vi "VAC_Measure_3.vi"() -> ()   [LabVIEW 2018]
doc: "Read one the value of one analog channel from a LINX device."
uses:
  <vilib>/MakerHub/LINX/Public/Peripherals/Digital/Digital Write N Chans.vi
  <vilib>/MakerHub/LINX/Public/Peripherals/Digital/Digital Write 1 Chan.vi
  <vilib>/MakerHub/LINX/Public/Peripherals/Analog/Analog Read N Chans.vi
  <vilib>/MakerHub/LINX/Private/Local IO/LinxDigitalWrite.vi
  <vilib>/MakerHub/LINX/Public/Utilities/Check Channel.vi
  <vilib>/MakerHub/LINX/Private/Local IO/LinxAnalogRead.vi
  <vilib>/MakerHub/LINX/Public/Utilities/Open Serial.vi
  <vilib>/MakerHub/LINX/Private/Utilties/Generate Error.vi
  <vilib>/MakerHub/LINX/LMH-LINX.lvlib
  LW/LIRA_toolbox.lvlib
panel:
  in  "Каналы разрядки":u8[](array[numeric])
  in  "Каналы зарядки":u8[](array[numeric])
  out "Напряжение":T1(graph)
  out "Ток":T1(graph)
  out "Напряжение":dbl[](array[numeric])
  out "Сила тока":dbl[](array[numeric])
  in  "Каналы чтения напряжения":u8[](array[numeric])
  in  "Каналы чтения тока":u8[](array[numeric])
  in  "Boolean":bool
  in  "Макс напряжение":dbl
  in  "Канал шторки":u8
  in  "Старт программы":bool
  in  "Напряжение":T2={"Измеряемая величина"="U", "единицы измерения"="В", "Ширина строки (в символах)"="16", "Количество знаков после запятой"="2"}
  in  "Сила тока":T2={"Измеряемая величина"="I", "единицы измерения"="A", "Ширина строки (в символах)"="16", "Количество знаков после запятой"="2"}
  in  "Количество стрингов":i32=1
  in  "Название файла":string="1"
  in  "Путь к файлу с указанием на случайный txt файл":path=path "I:/Снятие_ВАХ/log/20250902_16_09_1.txt"
  in  "Старт измерений":bool
  out "array of clusters":cluster{"Voltage":dbl, "Voltage":dbl}[](array[cluster])
  out "ВАХ":cluster{"X":dbl, "Y":dbl}[](graph)
  out "Loop Rate (Hz)":u32
  in  "Stop Button":bool
  in  "Serial Port":refnum<visa-resource-name>="COM6"
  # "Панель управления"
  # "LINX Device Settings"
  # "Панель вывода данных на экран"
  # "Панель вывода данных в файл"
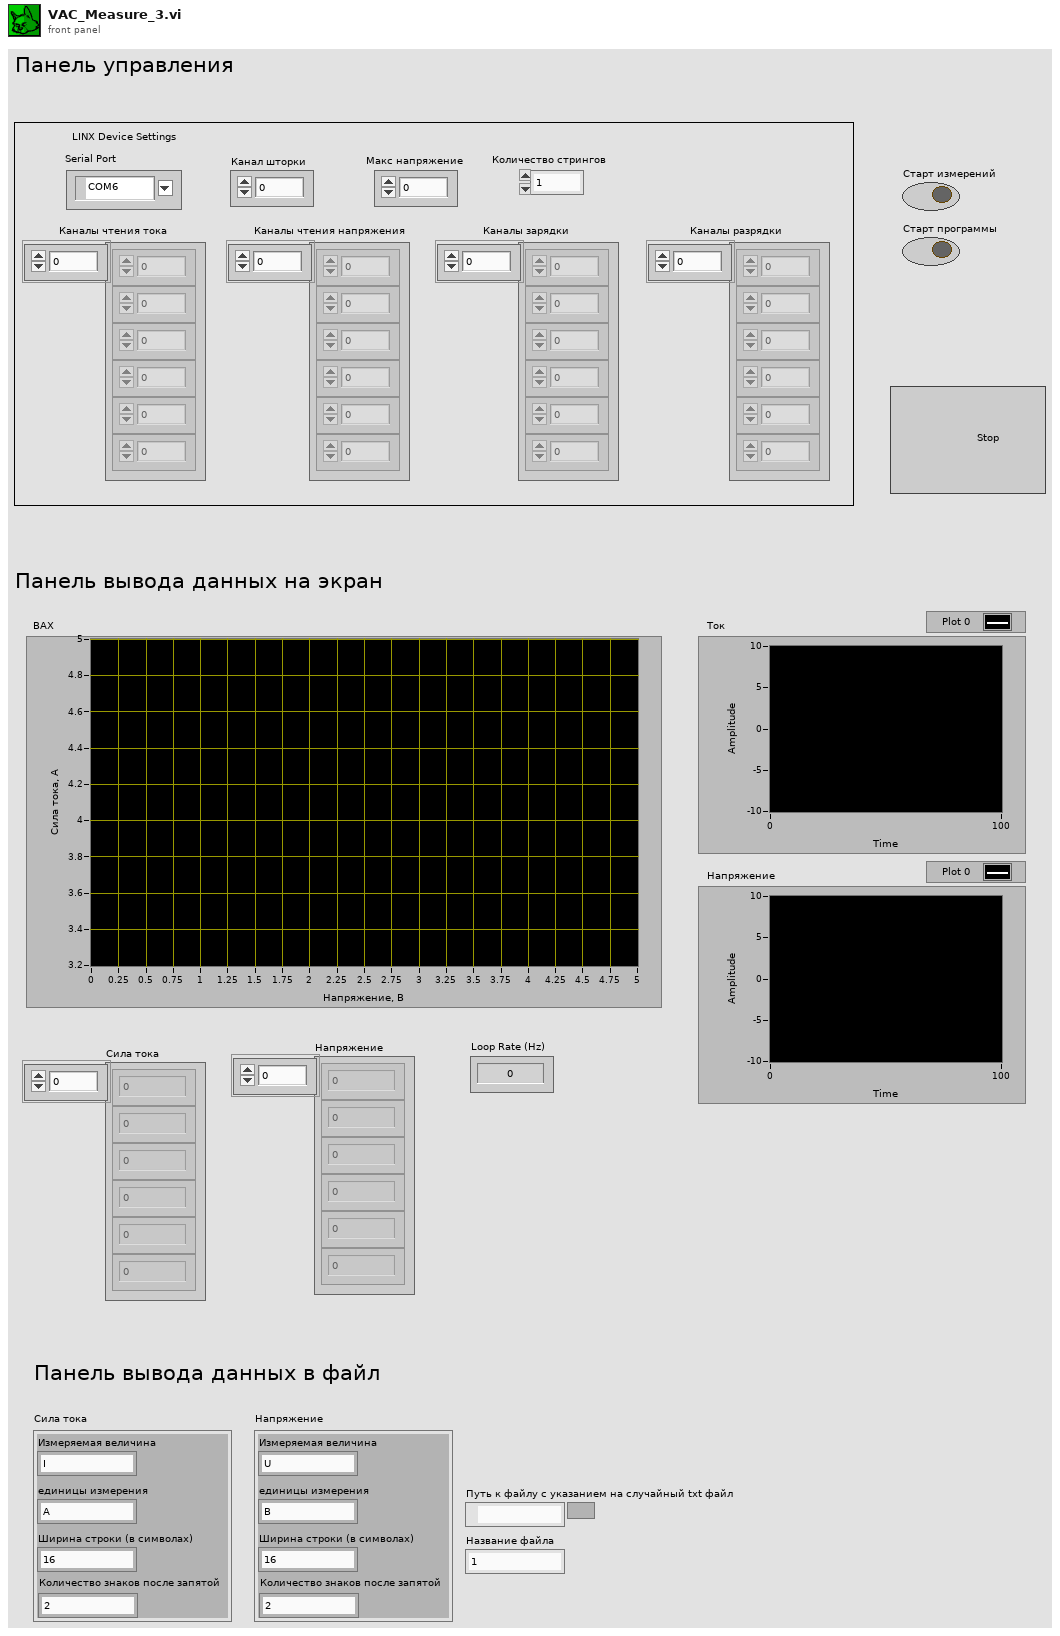
[diagram p1: front panel]
types:
  T1 = cluster{"Voltages[0]":dbl, "Voltages[1]":dbl, "Voltages[2]":dbl, "Voltages[3]":dbl, "Voltages[4]":dbl, "Voltages[5]":dbl, "Voltages[6]":dbl, "Voltages[7]":dbl, "Voltages[8]":dbl}
  T2 = cluster{"Измеряемая величина":string, "единицы измерения":string, "Ширина строки (в символах)":string, "Количество знаков после запятой":string}
  T3 = typedef "LMH-LINX.lvlib/LINX Ref.ctl" = cluster{"IO":T4, "Interface":T5, "LINX Device Config":T6}
  T4 = typedef "LMH-LINX.lvlib/Platform.ctl" = enum16{"Remote", "Local"}
  T5 = typedef "LMH-LINX.lvlib/Interface.ctl" = enum16{"Serial", "TCP"}
  T6 = typedef "LMH-LINX.lvlib/Device.lvlib/LINX Device Config.ctl" = cluster{"Interface":T5, "COM Port":refnum<visa-resource-name>, "TCP Configuration":T7, "Device Family":u8, "Device ID":u8, "Device Name":string, "TCP Ref":refnum<k5>, "Channels":T8}
  T7 = typedef "LMH-LINX.lvlib/Device.lvlib/TCP Config.ctl" = cluster{"IP Address":string, "Port":u16}
  T8 = typedef "LMH-LINX.lvlib/Channels.ctl" = cluster{"DI":u8[], "DO":u8[], "AI":u8[], "AO":u8[], "PWM":u8[], "QE":u8[], "UART":u8[], "I2C 2":u8[], "SPI":u8[], "CAN":u8[], "Servo":u8[], "AI Ref (V)":dbl, "AI Resolution (Bits)":u8, "AO Ref (V)":dbl, "AO Resolution (Bits)":u8}
  T9 = cluster{"Numeric Control":dbl, "Numeric Control":dbl}[]
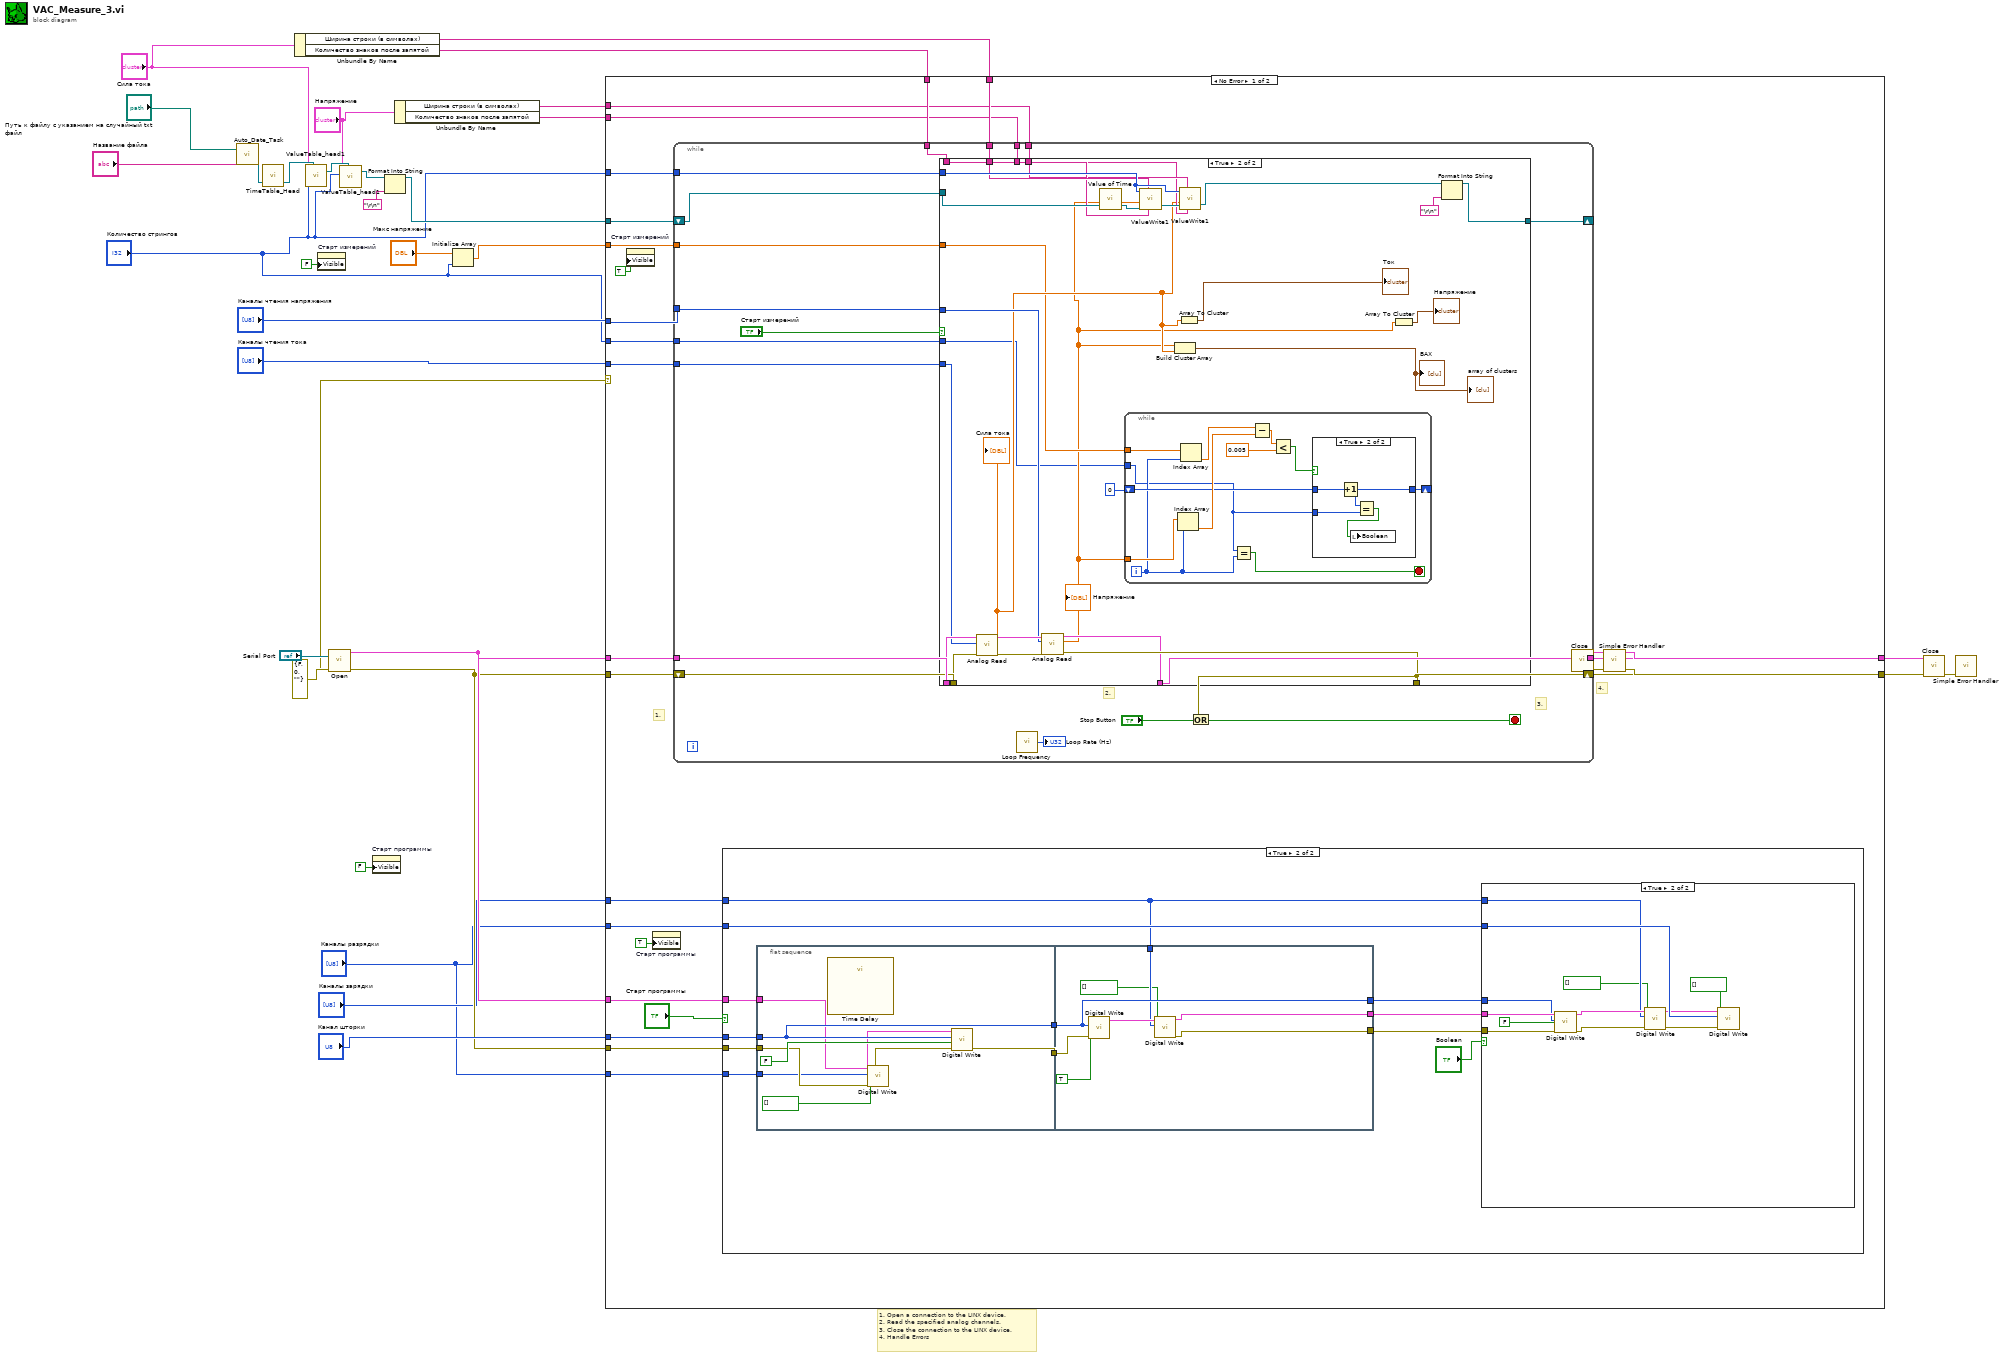
[diagram p0: block diagram]
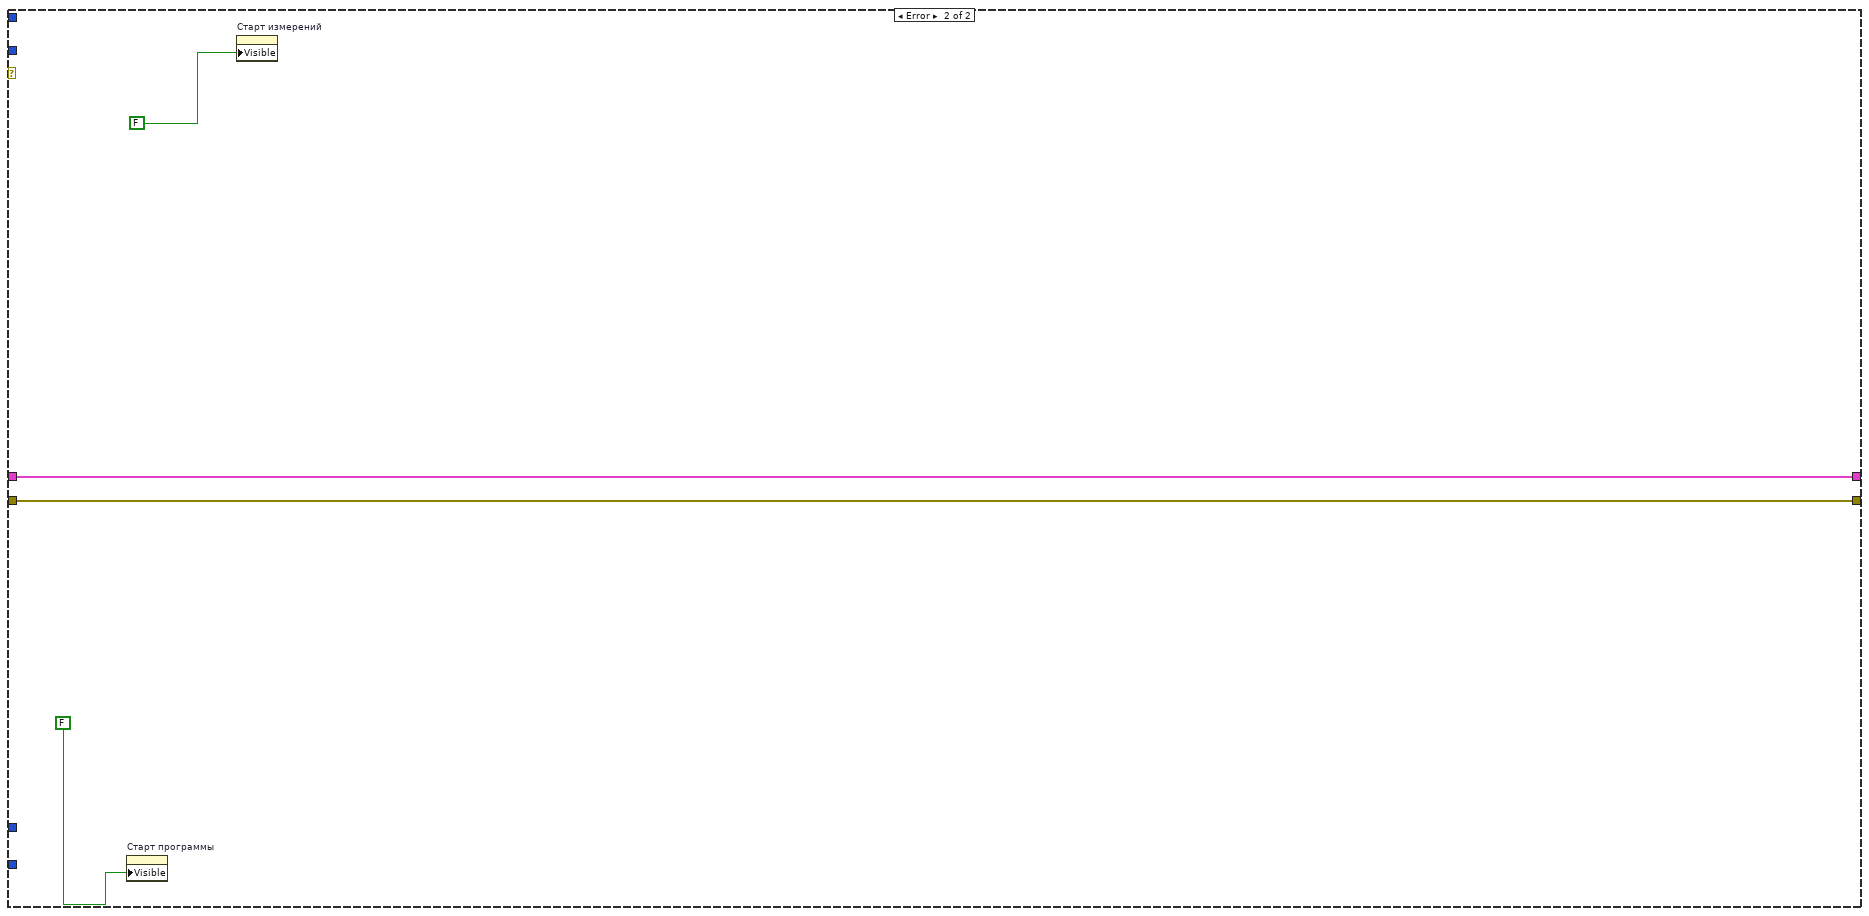
[diagram p6: hidden frame]
diagram:
  # "1. Open a connection to the LINX device.\n2. Read the specified analog channels.\n3. Close the connection to the LINX device.\n4. Handle Errors"
  # "4."
  n1 = call "Auto_Date_Task.vi"("Название файла"="Название файла", "Путь к файлу с указанием на случайный txt файл"="Путь к файлу с указанием на случайный txt файл") -> ("refnum out"=w26:refnum<file>)  [unwired: 1 out]
  n2 = call "TimeTable_Head.vi"("input file"=w26) -> ("output file refnum"=w25:refnum<file>)  [unwired: 1 in, 1 out]
  n3 = Unbundle By Name("Сила тока") -> ("Ширина строки (в символах)"=w22:string, "Количество знаков после запятой"=w21:string)
  n4 = call "ValueTable_head1.vi"("Файл записи"=w25, "Количество датчиков"="Количество стрингов", "Cluster"="Сила тока") -> ("Файл записи 2"=w24:refnum<file>)  [unwired: 3 in, 1 out]
  n5 = property on="Старт измерений" class="Bool (strict)"("Visible"=FALSE) -> ()  [unwired: 2 in, 2 out]
  n6 = call-poly <vilib>:"Open.vi"("Error In"=errorcluster {"status"=FALSE, "code"=0, "source"=""}, "Serial Port"="Serial Port") -> ("Error Out"=w11:errorcluster, "LINX Resource"=w13:T3)  [unwired: 7 in, 1 out]
  n7 = call "ValueTable_head1.vi"("Файл записи"=w24, "Количество датчиков"="Количество стрингов", "Cluster"="Напряжение") -> ("Файл записи 2"=w16:refnum<file>)  [unwired: 3 in, 1 out]
  n8 = property on="Старт программы" class="Bool (strict)"("Visible"=FALSE) -> ()  [unwired: 2 in, 2 out]
  n9 = Format Into String(initial string=w16, "\r\n") -> (resulting string=w15:refnum<file>)  [unwired: 2 in, 1 out]
  n10 = Unbundle By Name("Напряжение") -> ("Ширина строки (в символах)"=w19:string, "Количество знаков после запятой"=w18:string)
  n11 = Initialize Array("Макс напряжение", "Количество стрингов") -> (w7:dbl[])
  n12 = case shown="No Error" w11 {
    tunnel: w13 -> [w55 w165]
    tunnel: w11 -> [w54 w166]
    tunnel: [w53 w165] -> w3
    tunnel: [w52 w166] -> w2
    tunnel: w15 -> [w51 _]
    tunnel: "Количество стрингов" -> [w49 _]
    tunnel: w22 -> [w48 _]
    tunnel: w21 -> [w47 _]
    tunnel: w19 -> [w46 _]
    tunnel: w18 -> [w45 _]
    tunnel: w13 -> [w42 _]
    tunnel: "Канал шторки" -> [w41 _]
    tunnel: w11 -> [w40 _]
    tunnel: "Каналы чтения тока" -> [w39 _]
    tunnel: "Каналы чтения напряжения" -> [w38 _]
    tunnel: w7 -> [w37 _]
    tunnel: "Количество стрингов" -> [w36 _]
    tunnel: "Каналы зарядки" -> [w35 _]
    tunnel: "Каналы разрядки" -> [w34 _]
    tunnel: "Каналы разрядки" -> [w33 _]
    frame No Error {
      # "3."
      # "1."
      n13 = property on="Старт измерений" class="Bool (strict)"("Visible"=TRUE) -> ()  [unwired: 2 in, 2 out]
      n14 = property on="Старт программы" class="Bool (strict)"("Visible"=TRUE) -> ()  [unwired: 2 in, 2 out]
      n15 = while {
        tunnel: w55 -> [w102]
        tunnel: [w114] -> w53
        shift-right: [w113] -> w52
        shift-left: w54 -> [w101]
        shift-right: [w111] -> _
        shift-left: w51 -> [w109]
        tunnel: w49 -> [w108]
        tunnel: w48 -> [w107]
        tunnel: w47 -> [w106]
        tunnel: w46 -> [w105]
        tunnel: w45 -> [w104]
        tunnel: w39 -> [w100]
        tunnel: w38 -> [w99]
        tunnel: w37 -> [w98]
        tunnel: w36 -> [w97]
        stop <- w112 stop-if-true
        # "2."
        n16 = case shown="True" "Старт измерений" {
          tunnel: [w116 w143] -> w113
          tunnel: [w117 w142] -> w114
          tunnel: [w118 w131] -> w111
          tunnel: w109 -> [w118 w141]
          tunnel: w108 -> [_ w138]
          tunnel: w107 -> [_ w137]
          tunnel: w106 -> [_ w136]
          tunnel: w105 -> [_ w135]
          tunnel: w104 -> [_ w134]
          tunnel: w102 -> [w117 w130]
          tunnel: w101 -> [w116 w129]
          tunnel: w100 -> [_ w128]
          tunnel: w99 -> [_ w127]
          tunnel: w98 -> [_ w122]
          tunnel: w97 -> [_ w120]
          frame False {
          }
          frame True {
            n17 = call-poly <vilib>:"Analog Read.vi"("Error In"=w129, "AI Channel(s)"=w128, "LINX Resource"=w130) -> ("Error Out"=w145:errorcluster, "Voltages"=w125:dbl[], "LINX Resource"=w144:T3)  [unwired: 5 in, 1 out]
            "Сила тока" <- w125
            n18 = call-poly <vilib>:"Analog Read.vi"("Error In"=w145, "AI Channel(s)"=w127, "LINX Resource"=w144) -> ("Error Out"=w143:errorcluster, "Voltages"=w121:dbl[], "LINX Resource"=w142:T3)  [unwired: 5 in, 1 out]
            "Напряжение" <- w121
            n19 = call "Value of Time.vi"("input file"=w141) -> ("output file refnum"=w140:refnum<file>)  [unwired: 1 in, 1 out]
            n20 = while {
              tunnel: w122 -> [w155]
              tunnel: w121 -> [w153]
              tunnel: w120 -> [w147]
              shift-right: [w149] -> _
              shift-left: 0 -> [w150]
              i -> [w148]
              stop <- w146 stop-if-true
              n21 = Index Array(array=w153, index=w148) -> (element=w152:dbl)
              n22 = Index Array(array=w155, index=w148) -> (element=w154:dbl)
              n23 = Equal?(x=w147, y=w148) -> (x = y?=w146:bool)
              n24 = Subtract(x=w154, y=w152) -> (x-y=w157:dbl)
              n25 = Less?(x=w157, y=0.005) -> (x < y?=w151:bool)
              n26 = case shown="True" w151 {
                tunnel: w147 -> [_ w162]
                tunnel: w150 -> [w158 w160]
                tunnel: [w158 w159] -> w149
                frame False {
                }
                frame True {
                  n27 = Increment(x=w160) -> (x+1=w159:i32)
                  n28 = Equal?(x=w159, y=w162) -> (x = y?=w161:bool)
                  n29 = local write "Boolean"(w161) -> ()
                }
              }
            }
            n30 = call "ValueWrite1.vi"("Количество знаков после запятой"=w136, "Ширина строки (в символах)"=w137, "Файл с заголовком"=w140, "Массив с измерениями"=w121, "Количество датчиков"=w138) -> ("Файл с заголовком 2"=w139:refnum<file>)  [unwired: 1 in, 1 out]
            n31 = Build Cluster Array(w121, w125) -> (→"ВАХ" →"array of clusters":T9)
            n32 = Array To Cluster(array=w125) -> (cluster=→"Ток":T1)
            n33 = call "ValueWrite1.vi"("Количество знаков после запятой"=w134, "Ширина строки (в символах)"=w135, "Файл с заголовком"=w139, "Массив с измерениями"=w125, "Количество датчиков"=w138) -> ("Файл с заголовком 2"=w132:refnum<file>)  [unwired: 1 in, 1 out]
            n34 = Array To Cluster(array=w121) -> (cluster=→"Напряжение":T1)
            n35 = Format Into String(initial string=w132, "\r\n") -> (resulting string=w131:refnum<file>)  [unwired: 2 in, 1 out]
          }
        }
        n36 = call <vilib>:"Loop Frequency.vi"() -> ("Loop Rate (Hz)"=→"Loop Rate (Hz)":u32)
        n37 = Or(x=w113, y="Stop Button") -> (x .or. y?=w112:bool)
      }
      n38 = case shown="True" "Старт программы" {
        tunnel: w42 -> [_ w67]
        tunnel: w41 -> [_ w66]
        tunnel: w40 -> [_ w65]
        tunnel: w35 -> [_ w57]
        tunnel: w34 -> [_ w58]
        tunnel: w33 -> [_ w56]
        frame False {
        }
        frame True {
          n39 = flat-sequence {
            tunnel: w67 -> [w85]
            tunnel: w66 -> [w87]
            tunnel: w65 -> [w83]
            tunnel: [w87] -> w64
            tunnel: [w86] -> w63
            tunnel: w56 -> [w81]
            tunnel: w64 -> [w91]
            tunnel: w63 -> [w96]
            tunnel: [w93] -> w61
            tunnel: [w92] -> w60
            tunnel: [w91] -> w59
            tunnel: w57 -> [w90]
            frame #0 {
              n40 = call "Time Delay"() -> ()  [unwired: 11 in, 1 out]
              n41 = call-poly <vilib>:"Digital Write.vi"("Error In"=w83, "Values"=bool[] [], "DO Channels"=w81, "LINX Resource"=w85) -> ("Error Out"=w82:errorcluster, "LINX Resource"=w84:T3)  [unwired: 6 in]
              n42 = call-poly <vilib>:"Digital Write.vi"("Error In"=w82, "Output Value"=FALSE, "DO Channel"=w87, "LINX Resource"=w84) -> ("Error Out"=w86:errorcluster)  [unwired: 6 in, 1 out]
            }
            frame #1 {
              n43 = call-poly <vilib>:"Digital Write.vi"("Error In"=w96, "Output Value"=TRUE, "DO Channel"=w91) -> ("LINX Resource"=w94:T3)  [unwired: 7 in, 1 out]
              n44 = call-poly <vilib>:"Digital Write.vi"("Values"=bool[] [], "DO Channels"=w90, "LINX Resource"=w94) -> ("Error Out"=w92:errorcluster, "LINX Resource"=w93:T3)  [unwired: 7 in]
            }
          }
          n45 = case shown="True" "Boolean" {
            tunnel: w61 -> [_ w79]
            tunnel: w60 -> [_ w78]
            tunnel: w59 -> [_ w77]
            tunnel: w58 -> [_ w74]
            tunnel: w57 -> [_ w69]
            frame False {
            }
            frame True {
              n46 = call-poly <vilib>:"Digital Write.vi"("Error In"=w78, "Output Value"=FALSE, "DO Channel"=w77, "LINX Resource"=w79) -> ("Error Out"=w71:errorcluster, "LINX Resource"=w73:T3)  [unwired: 6 in]
              n47 = call-poly <vilib>:"Digital Write.vi"("Error In"=w71, "Values"=bool[] [], "DO Channels"=w69, "LINX Resource"=w73) -> ("Error Out"=w70:errorcluster, "LINX Resource"=w72:T3)  [unwired: 6 in]
              n48 = call-poly <vilib>:"Digital Write.vi"("Error In"=w70, "Values"=bool[] [], "DO Channels"=w74, "LINX Resource"=w72) -> ()  [unwired: 6 in, 2 out]
            }
          }
        }
      }
    }
    frame Error {
      n49 = property on="Старт программы" class="Bool (strict)"("Visible"=FALSE) -> ()  [unwired: 2 in, 2 out]
      n50 = property on="Старт измерений" class="Bool (strict)"("Visible"=FALSE) -> ()  [unwired: 2 in, 2 out]
    }
  }
  n51 = call <vilib>:"Close.vi"("Error In"=w2, "LINX Resource"=w3) -> ("Error Out"=w31:errorcluster)  [unwired: 9 in]
  n52 = call <vilib>:"Simple Error Handler.vi"("error in (no error)"=w31) -> ()  [unwired: 4 in, 5 out]
  n53 = call <vilib>:"Close.vi"("Error In"=w2, "LINX Resource"=w3) -> ("Error Out"=w1:errorcluster)  [unwired: 9 in]
  n54 = call <vilib>:"Simple Error Handler.vi"("error in (no error)"=w1) -> ()  [unwired: 4 in, 5 out]
